vi "Rotate 3D object LV2012.vi"() -> ()   [LabVIEW 2012]
uses:
  <vilib>/picture/3D Picture Control/NI_3D Picture Control.lvlib
  <vilib>/picture/3D Picture Control/Object/Create Object (name).vi
panel:
  in  "Right":bool
  in  "Left":bool
  in  "Clockwise":bool
  in  "Counter Clockwise":bool
  in  "stop":bool
  out "3D Picture":refnum<vi>(3d-picture)
  in  "Up":bool
  in  "Down":bool
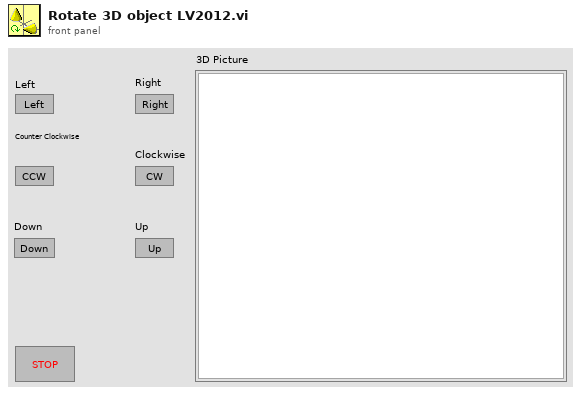
[diagram p1: front panel]
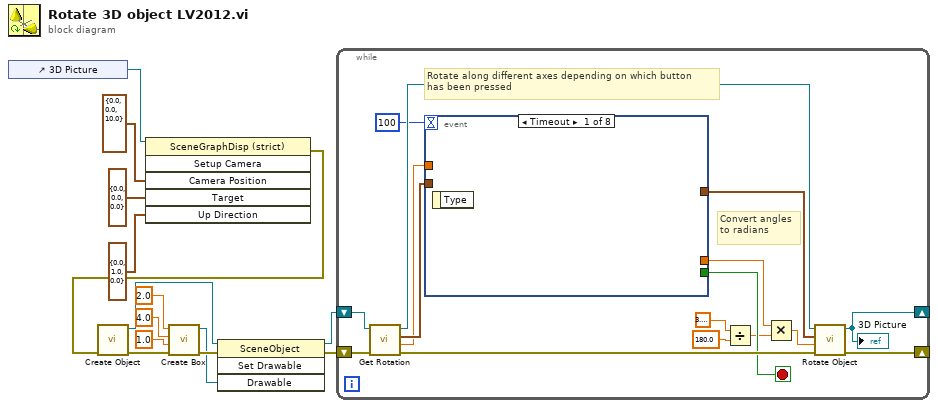
[diagram p0: block diagram]
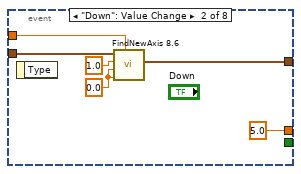
[diagram p2: hidden frame]
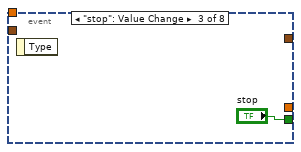
[diagram p3: hidden frame]
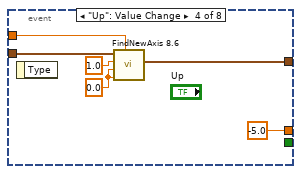
[diagram p4: hidden frame]
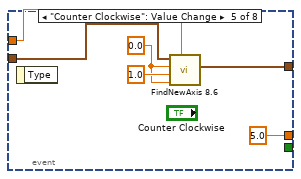
[diagram p5: hidden frame]
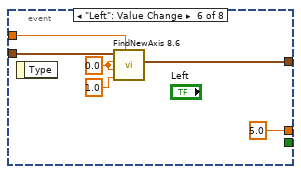
[diagram p6: hidden frame]
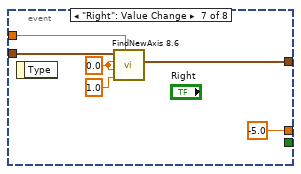
[diagram p7: hidden frame]
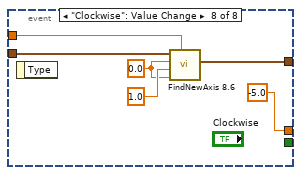
[diagram p8: hidden frame]
diagram:
  n1 = control-ref of="3D Picture"() -> (w2:refnum<vi>)
  n2 = invoke on="Invoke Node" class="SceneGraphDisp (strict)" method="Setup Camera"(reference=w2, "Camera Position"=cluster{"X":sgl, "Y":sgl, "Z":sgl} {"X"=0.0, "Y"=0.0, "Z"=10.0}, "Target"=cluster{"X":sgl, "Y":sgl, "Z":sgl} {"X"=0.0, "Y"=0.0, "Z"=0.0}, "Up Direction"=cluster{"X":sgl, "Y":sgl, "Z":sgl} {"X"=0.0, "Y"=1.0, "Z"=0.0}) -> (error out=w1:errorcluster)  [unwired: 2 in, 5 out]
  n3 = call-poly <vilib>:"Create Object.vi"("error in (no error)"=w1) -> ("error out"=w5:errorcluster, "Scene:New Object"=w11:refnum<vi>)  [unwired: 9 in]
  n4 = call <vilib>:"Create Box.vi"("error in (no error)"=w5, "Length Z"=sgl 1.0, "Length Y"=sgl 4.0, "Length X"=sgl 2.0) -> ("error out"=w4:errorcluster, "New Box Refnum"=w3:refnum<vi>)  [unwired: 6 in]
  n5 = invoke class="SceneObject" method="Set Drawable"(reference=w11, error in=w4, "Drawable"=w3) -> (reference out=w10:refnum<vi>, error out=w9:errorcluster)  [unwired: 1 in, 2 out]
  n6 = while {
    shift-right: [w22] -> _
    shift-left: w10 -> [w30]
    shift-right: [w21] -> _
    shift-left: w9 -> [w29]
    stop <- w26 stop-if-true
    # "Convert angles\nto radians"
    # "Rotate along different axes depending on which button\nhas been pressed"
    n7 = call <vilib>:"Get Rotation.vi"("error in (no error)"=w29, "Scene Object"=w30) -> ("error out"=w27:errorcluster, "Angle"=w24:sgl, "Axis"=w25:cluster{"X":sgl, "Y":sgl, "Z":sgl}, "Scene Object"=w28:refnum<vi>)  [unwired: 6 in]
    n8 = event shown="[0] Timeout" {
      selector: _ -> [_ _ _ _ _ _ _ _]
      dyn-events: _ -> [_ _ _ _ _ _ _ _]
      timeout: 100 -> [_ _ _ _ _ _ _ _]
      tunnel: [_ sgl 5.0 ("Angle") _ sgl -5.0 ("Angle") sgl 5.0 ("Angle") sgl 5.0 ("Angle") sgl -5.0 ("Angle") sgl -5.0 ("Angle")] -> w20
      tunnel: [_ _ "stop" _ _ _ _ _] -> w26
      tunnel: w25 -> [_ w32 _ w42 w48 w54 w60 w66]
      tunnel: w24 -> [_ w33 _ w41 w47 w53 w59 w65]
      tunnel: [_ w31 _ w38 w46 w52 w58 w64] -> w23
      event Timeout {
        n9 = event-data() -> ()  [unwired: 1 in, 1 out]
      }
      event "Down": Value Change {
        w34 = 0.0 ("Z")
        n10 = event-data() -> ()  [unwired: 1 in, 1 out]
        n11 = call "FindNewAxis 8.6.vi"("Angle"=w33, "Y"=w34, "Z"=w34, "X"=1.0, "Axis"=w32) -> ("New Axis"=w31:cluster{"X":sgl, "Y":sgl, "Z":sgl})  [unwired: 4 in]
      }
      event "stop": Value Change {
        n12 = event-data() -> ()  [unwired: 1 in, 1 out]
      }
      event "Up": Value Change {
        w39 = 0.0 ("Z")
        n13 = event-data() -> ()  [unwired: 1 in, 1 out]
        n14 = call "FindNewAxis 8.6.vi"("Angle"=w41, "Y"=w39, "Z"=w39, "X"=1.0, "Axis"=w42) -> ("New Axis"=w38:cluster{"X":sgl, "Y":sgl, "Z":sgl})  [unwired: 4 in]
      }
      event "Counter Clockwise": Value Change {
        w44 = 0.0 ("Z")
        n15 = event-data() -> ()  [unwired: 1 in, 1 out]
        n16 = call "FindNewAxis 8.6.vi"("Angle"=w47, "Y"=w44, "Z"=1.0 ("X"), "X"=w44, "Axis"=w48) -> ("New Axis"=w46:cluster{"X":sgl, "Y":sgl, "Z":sgl})  [unwired: 4 in]
      }
      event "Left": Value Change {
        w50 = 0.0 ("Z")
        n17 = event-data() -> ()  [unwired: 1 in, 1 out]
        n18 = call "FindNewAxis 8.6.vi"("Angle"=w53, "Y"=1.0 ("X"), "Z"=w50, "X"=w50, "Axis"=w54) -> ("New Axis"=w52:cluster{"X":sgl, "Y":sgl, "Z":sgl})  [unwired: 4 in]
      }
      event "Right": Value Change {
        w56 = 0.0 ("Z")
        n19 = event-data() -> ()  [unwired: 1 in, 1 out]
        n20 = call "FindNewAxis 8.6.vi"("Angle"=w59, "Y"=1.0 ("X"), "Z"=w56, "X"=w56, "Axis"=w60) -> ("New Axis"=w58:cluster{"X":sgl, "Y":sgl, "Z":sgl})  [unwired: 4 in]
      }
      event "Clockwise": Value Change {
        w62 = 0.0 ("Z")
        n21 = event-data() -> ()  [unwired: 1 in, 1 out]
        n22 = call "FindNewAxis 8.6.vi"("Angle"=w65, "Y"=w62, "Z"=1.0 ("X"), "X"=w62, "Axis"=w66) -> ("New Axis"=w64:cluster{"X":sgl, "Y":sgl, "Z":sgl})  [unwired: 4 in]
      }
    }
    n23 = Divide(x=3.141592653589793, y=180.0) -> (x/y=w16:dbl)
    n24 = Multiply(x=w20, y=w16) -> (x*y=w19:dbl)
    n25 = call <vilib>:"Rotate Object.vi"("error in (no error)"=w27, "Angle"=w19, "Axis"=w23, "Scene.Object In"=w28) -> ("error out"=w21:errorcluster, "Scene.Object Out"=w22:refnum<vi>)  [unwired: 6 in]
    "3D Picture" <- w22
  }
